vi "CNT90_main.vi"() -> ()   [LabVIEW 2019]
doc: "This example shows how to use autosetup and acquire a result of frequency on a single channel for acquiring results in a loop until stopped by user."
uses:
  <vilib>/Utility/file.llb/Write Delimited Spreadsheet (string).vi
  CNT90_share/Pendulum CNT90-simple/Pendulum CNT90/Public/Data/Read Measurement (Single).vi
  <vilib>/Utility/file.llb/Write Delimited Spreadsheet (DBL).vi
  CNT90_share/Pendulum CNT90-simple/Pendulum CNT90/Pendulum CNT90.lvlib
panel:
  out "?":T1
  out "Filepath (will be \\data in this VI directory, and \nmade to match Moku data .csv's)":path
  out "Time elapsed [s]":dbl
  in  "Loop time [ms]":i64=350
  in  "Write to File?":bool=TRUE
  out "Running?":bool
  out "Error Out":errorcluster
  out "Meas. #":i32
  out "Start Time":timestamp
  out "Freq. Chart":dbl(graph)
  in  "Gate Time [s]":dbl=0.1
  in  "Channel  2 (0: A)":i32(ring) items=["A", "B", "C (HF-input option)", "E (Rear panel arming input)", "A prescaled by 2", "Internal Reference", "A with the variable hysteresis mode"]
  in  "Channel  1 (0: A)":i32(ring) items=["A", "B", "C (HF-input option)", "E (Rear panel arming input)", "A prescaled by 2", "Internal Reference", "A with the variable hysteresis mode"]
  in  "Stop":bool
  out "Last read [Hz]":dbl format="%#_16f"
  in  "Timeout [ms]":i32=1000
  in  "VISA resource name":refnum<visa-resource-name>
  # "Paul Edwards\n2022-Dec.\n___________________________________________\nSingle channel, constant freq. acquisition for CNT-90 freq. counter.\n\nCNT-90 driver version: 2.1\nLabVIEW 2019"
  # "CNT-90 Manuals\n____________________\nGeneral: https://pendulum-instruments.com/wp-content/uploads/2022/05/CNT-90_91um_Rev22-1.pdf\n\nProgammers: https://pendulum-instruments.com/wp-content/uploads/2022/05/CNT-90ph-1.pdf"
  # "Frequency Data"
  # "Counter Setup"
  # "Setup Output Files (.csv)"
  # "Misc. Data"
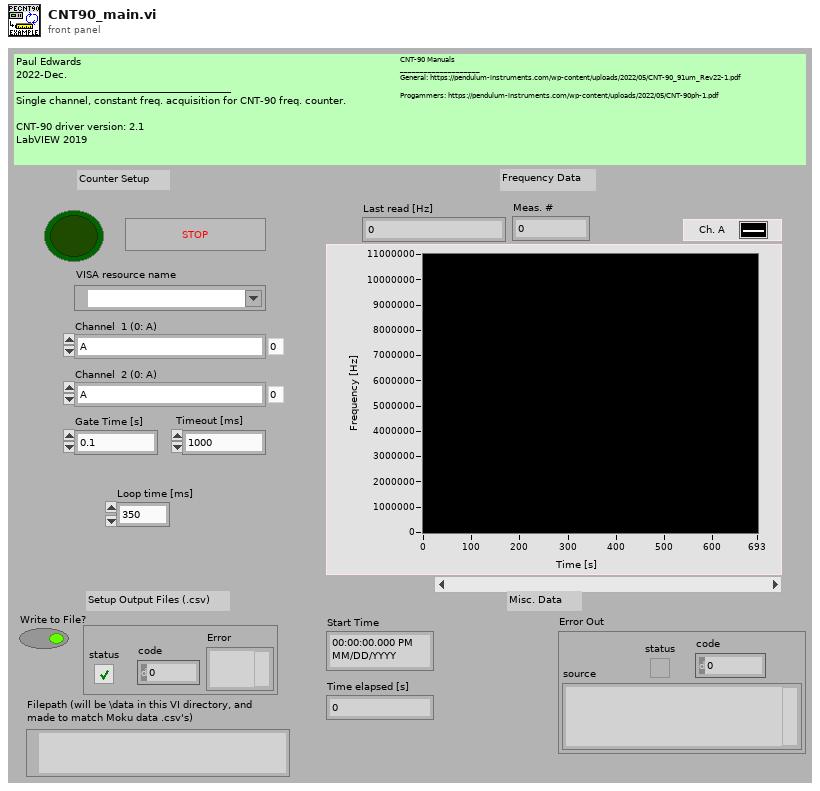
[diagram p1: front panel]
types:
  T1 = cluster{"status":bool, "code":i32, "Error":string}
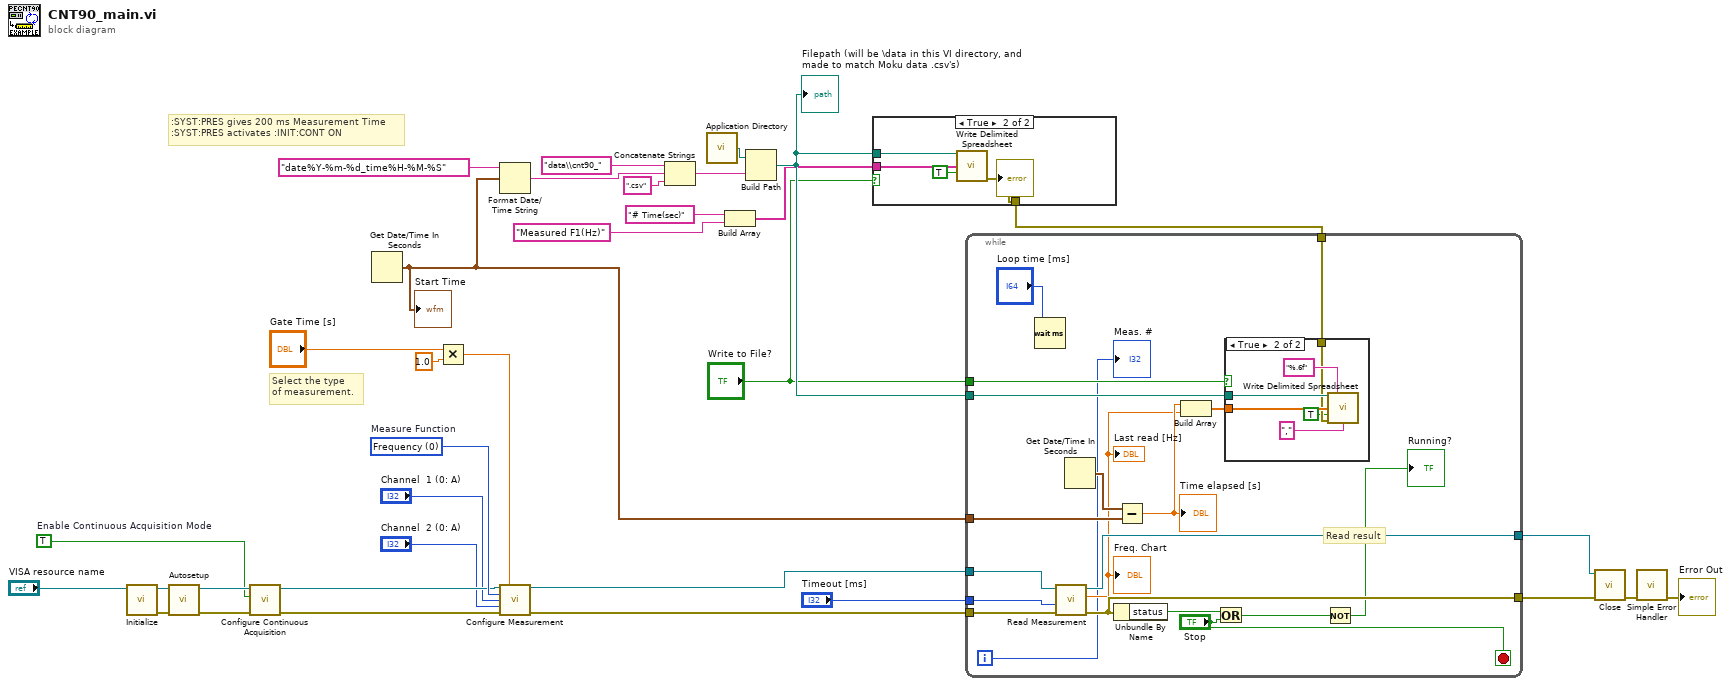
[diagram p0: block diagram]
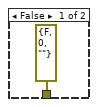
[diagram p3: hidden frame]
diagram:
  w20 = TRUE  # Enable Continuous Acquisition Mode
  w25 = 0 items=["Frequency", "Burst Carrier Frequency", "Pulse Repetition Frequency", "Fall-time", "Frequency Ratio", "Positive Peak Voltage", "Negative Peak Voltage", "Negative Pulse Width", "Positive Pulse Width", "Positive Duty Cycle", "Negative Duty Cycle", "Phase", "Period", "Rise-time", "Peak-to-Peak Voltage", "Time-Interval"]  # Measure Function
  # ":SYST:PRES gives 200 ms Measurement Time\n:SYST:PRES activates :INIT:CONT ON"
  # "Select the type\nof measurement."
  n1 = call "Initialize.vi"("VISA resource name"="VISA resource name") -> ("error out"=w28:errorcluster, "VISA resource name out"=w29:refnum<visa-resource-name>)  [unwired: 9 in]
  n2 = call "Autosetup.vi"("error in (no error)"=w28, "VISA resource name"=w29) -> ("error out"=w23:errorcluster, "VISA resource name out"=w24:refnum<visa-resource-name>)  [unwired: 8 in]
  n3 = call "Configure Continuous Acquisition.vi"("error in (no error)"=w23, "Enable Continuous Acquisition Mode (T: True)"=w20, "VISA resource name"=w24) -> ("error out"=w21:errorcluster, "VISA resource name out"=w22:refnum<visa-resource-name>)  [unwired: 7 in]
  n4 = Get Date/Time In Seconds() -> (seconds since 1Jan1904=w5:timestamp)
  "Start Time" <- w5
  n5 = Multiply(x="Gate Time [s]", y=1.0) -> (x*y=w15:dbl)
  n6 = Format Date/Time String(time format string (%c)="date%Y-%m-%d_time%H-%M-%S", seconds (now)=w5) -> (date/time string=w13:string)  [unwired: 1 in]
  n7 = call "Configure Measurement.vi"("VISA resource name"=w22, "Measurement Time (0.01)"=w15, "Measure Function (0: Frequency)"=w25, "Channel  1 (0: A)"="Channel  1 (0: A)", "Channel  2 (0: A)"="Channel  2 (0: A)", "error in (no error)"=w21) -> ("VISA resource name out"=w27:refnum<visa-resource-name>, "error out"=w26:errorcluster)  [unwired: 8 in]
  n8 = Concatenate Strings("data\\cnt90_", w13, ".csv") -> (w7:string)
  n9 = call <vilib>:"Application Directory.vi"() -> ("Application Directory"=w6:path)
  n10 = Build Array("# Time(sec)", "Measured F1(Hz)") -> (w3:string[])
  n11 = Build Path(base path=w6, name or relative path=w7) -> (appended path=w4:path)
  "Filepath (will be \\data in this VI directory, and \nmade to match Moku data .csv's)" <- w4
  n12 = case shown="True" "Write to File?" {
    tunnel: w4 -> [_ w39]
    tunnel: w3 -> [_ w38]
    tunnel: [errorcluster {"status"=FALSE, "code"=0, "source"=""} ("error out") w37] -> w1
    frame False {
    }
    frame True {
      n13 = call-poly <vilib>:"Write Delimited Spreadsheet.vi"("file path (dialog if empty)"=w39, "1D data"=w38, "append to file? (new file:F)"=TRUE) -> ("error out"=w37:errorcluster)  [unwired: 11 in, 1 out]
      "?" <- w37
    }
  }
  n14 = while {
    tunnel: [w58] -> w33
    tunnel: [w57] -> w32
    tunnel: "Timeout [ms]" -> [w56]
    tunnel: w27 -> [w55]
    tunnel: w26 -> [w54]
    tunnel: "Write to File?" -> [w53]
    tunnel: w5 -> [w52]
    tunnel: w4 -> [w51]
    tunnel: w1 -> [w50]
    i -> [w42]
    stop <- "Stop" stop-if-true
    # "Read result"
    n15 = Wait (ms)(milliseconds to wait="Loop time [ms]") -> ()  [unwired: 1 out]
    n16 = call-poly "Read Measurement.vi"("error in (no error)"=w54, "Timeout (10000 ms)"=w56, "VISA resource name"=w55) -> ("error out"=w57:errorcluster, "Measurement"=w44:dbl, "VISA resource name out"=w58:refnum<visa-resource-name>)  [unwired: 6 in]
    "Last read [Hz]" <- w44
    "Freq. Chart" <- w44
    n17 = Get Date/Time In Seconds() -> (seconds since 1Jan1904=w46:timestamp)
    n18 = Unbundle By Name(w57) -> ("status"=w49:bool)
    n19 = Subtract(x=w46, y=w52) -> (x-y=w45:dbl)
    "Time elapsed [s]" <- w45
    n20 = Build Array(w45, w44) -> (w43:dbl[])
    n21 = Or(x=w49, y="Stop") -> (x .or. y?=w48:bool)
    n22 = case shown="True" w53 {
      tunnel: w51 -> [_ w62]
      tunnel: w43 -> [_ w61]
      tunnel: w50 -> [_ w60]
      frame False {
      }
      frame True {
        n23 = call-poly <vilib>:"Write Delimited Spreadsheet.vi"("file path (dialog if empty)"=w62, "format (%.3f)"="%.6f", "1D data"=w61, "append to file? (new file:F)"=TRUE, "error in (no error)"=w60, "delimiter (\\t)"="," ("delimiter (\\t)")) -> ()  [unwired: 8 in, 2 out]
      }
    }
    n24 = Not(x=w48) -> (.not. x?=→"Running?":bool)
    "Meas. #" <- w42
  }
  n25 = call "Close.vi"("error in (no error)"=w32, "VISA resource name"=w33) -> ("error out"=w34:errorcluster)  [unwired: 9 in]
  n26 = call <vilib>:"Simple Error Handler.vi"("error in (no error)"=w34) -> ("error out"=→"Error Out":errorcluster)  [unwired: 4 in, 4 out]
